vi "PM100-Set Range.vi"(0 "VISA in":refnum<visa-resource-name>, 7 "Autoscale?":bool, 9 "Range index":u16, 11 "error in (no error)":errorcluster) -> (4 "VISA out":refnum<visa-resource-name>, 15 "error out":errorcluster)   [LabVIEW 2015]
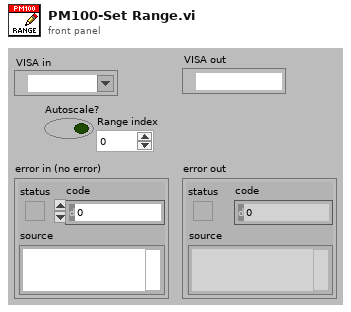
[diagram p1: front panel]
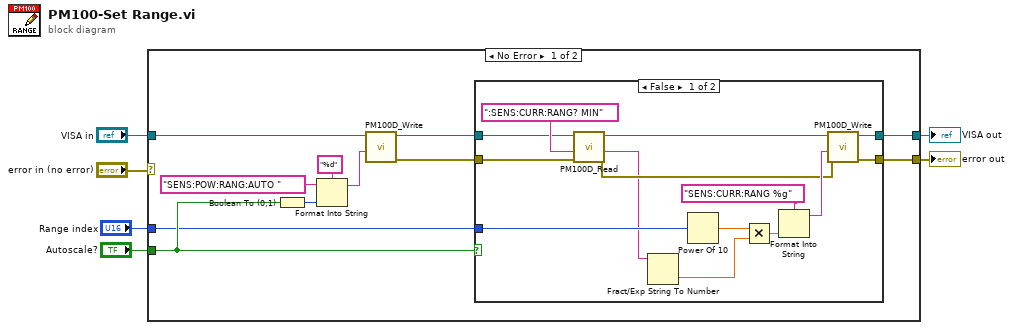
[diagram p0: block diagram]
diagram:
  n1 = case shown="No Error" "error in (no error)" {
    selector: "error in (no error)" -> [_ w34]
    tunnel: "VISA in" -> [w17 w35]
    tunnel: "Autoscale?" -> [w10 _]
    tunnel: [w7 w35] -> w3
    tunnel: [w8 w34] -> w2
    tunnel: "Range index" -> [w9 _]
    frame No Error {
      n2 = Boolean To (0,1)(Boolean=w10) -> (0, 1=w16:i16)
      n3 = Format Into String(format string="%d", initial string="SENS:POW:RANG:AUTO " ("Command"), w16) -> (resulting string=w13:string)  [unwired: 1 in, 1 out]
      n4 = call "PM100D_Write.vi"("Command"=w13, "VISA in"=w17) -> ("error out"=w11:errorcluster, "VISA out"=w12:refnum<visa-resource-name>)  [unwired: 8 in]
      n5 = case shown="False" w10 {
        tunnel: w12 -> [w24 w33]
        tunnel: w11 -> [w23 w32]
        tunnel: w9 -> [w22 _]
        tunnel: [w21 w32] -> w8
        tunnel: [w20 w33] -> w7
        frame False {
          n6 = call "PM100D_Read.vi"("error in (no error)"=w23, "Command"=":SENS:CURR:RANG? MIN", "VISA in"=w24) -> ("error out"=w28:errorcluster, "ReadValue"=w19:string, "VISA out"=w30:refnum<visa-resource-name>)  [unwired: 6 in]
          n7 = Fract/Exp String To Number(string=w19) -> (number=w29:dbl)  [unwired: 3 in, 1 out]
          n8 = Power Of 10(x=w22) -> (10^x=w26:dbl)
          n9 = Multiply(x=w26, y=w29) -> (x*y=w18:dbl)
          n10 = Format Into String(format string="SENS:CURR:RANG %g" ("Command"), w18) -> (resulting string=w31:string)  [unwired: 2 in, 1 out]
          n11 = call "PM100D_Write.vi"("error in (no error)"=w28, "Command"=w31, "VISA in"=w30) -> ("error out"=w21:errorcluster, "VISA out"=w20:refnum<visa-resource-name>)  [unwired: 7 in]
        }
        frame True {
        }
      }
    }
    frame Error {
    }
  }
  "error out" <- w2
  "VISA out" <- w3
